vi "Add Aggregate Log.vi"(8 "error in (no error)":errorcluster, 10 "Aggregate Enqueuer":refnum<queue>, 11 "LoggerReference in":refnum<class "LoggerReference.lvclass">) -> (0 "error out":errorcluster, 3 "LoggerReference out":refnum<class "LoggerReference.lvclass">)   [LabVIEW 2018, in "MVA Framework.lvlib" / "Composed Log.lvlib" / "LoggerReference.lvclass"]
uses:
  LoggerReference.lvclass
  Types/MessageCluster.ctl
  Composed Log.lvlib
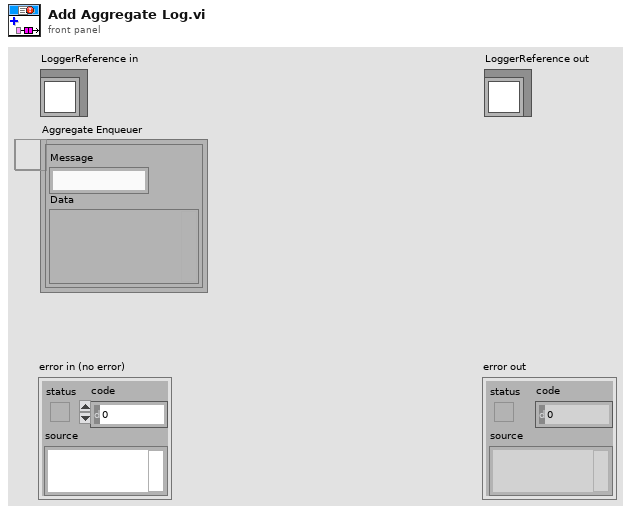
[diagram p1: front panel]
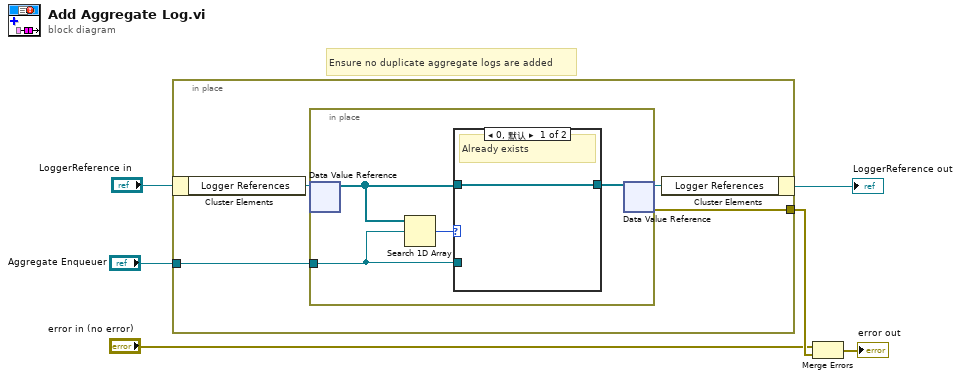
[diagram p0: block diagram]
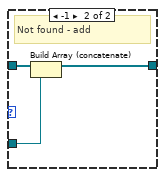
[diagram p2: hidden frame]
diagram:
  # "Ensure no duplicate aggregate logs are added"
  n1 = in-place {
    in-place-border: "Aggregate Enqueuer" -> [w10]
    in-place-border: [w7] -> w4
    n2 = in-place-cluster #1("LoggerReference in") -> ("Logger References"=w9:refnum<data-value>)
    n3 = in-place {
      in-place-border: w10 -> [w12]
      n4 = in-place-dvr #2(w9) -> (w11:refnum<queue>[])  [unwired: 1 out]
      n5 = Search 1D Array(1D array=w11, element=w12) -> (index of element=w14:i32)  [unwired: 1 in]
      n6 = case shown="0, 默认" w14 {
        tunnel: w11 -> [w15 w18]
        tunnel: w12 -> [_ w16]
        tunnel: [w15 w17] -> w13
        frame 0, Default {
          # "Already exists"
        }
        frame -1 {
          # "Not found - add"
          n7 = Build Array (concatenate)(w18, w16) -> (w17:refnum<queue>[])
        }
      }
      n8 = in-place-dvr #2(w13) -> (w8:refnum<data-value>, w7:errorcluster)
    }
    n9 = in-place-cluster #1("Logger References"=w8) -> (→"LoggerReference out":refnum<class "LoggerReference.lvclass">)
  }
  n10 = Merge Errors("error in (no error)", w4) -> (→"error out":errorcluster)
